vi "Test_WriteValue_InvalidType_Error.vi"(8 "error in (no error)":errorcluster, 11 "TestCase in":refnum<class "TestTerminalVisibilityBinding.lvclass">) -> (0 "error out":errorcluster, 3 "TestCase out":refnum<class "TestTerminalVisibilityBinding.lvclass">)   [LabVIEW 2017, in "TestTerminalVisibilityBinding.lvclass"]
uses:
  TestTerminalVisibilityBinding.lvclass
  Source/Concrete/TerminalVisibilityBinding/TerminalVisibilityBinding.lvclass
  C:/Git/composed-transport/Source/ITransport/ITransport.lvclass
  Source/ITransport/ITransport.lvclass
panel:
  in  "Numeric":dbl
  out "Return Error":errorcluster
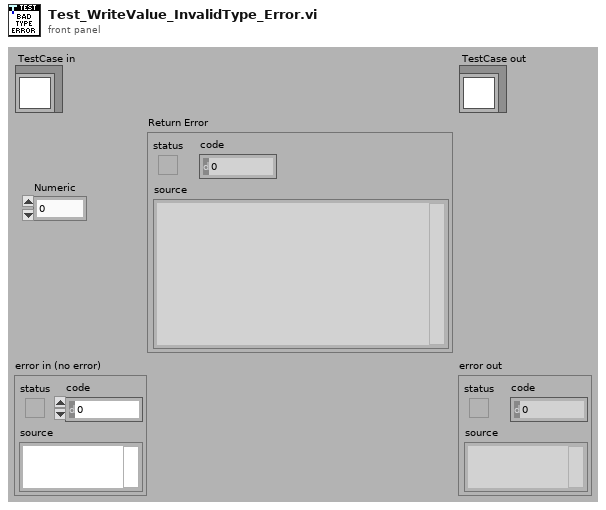
[diagram p1: front panel]
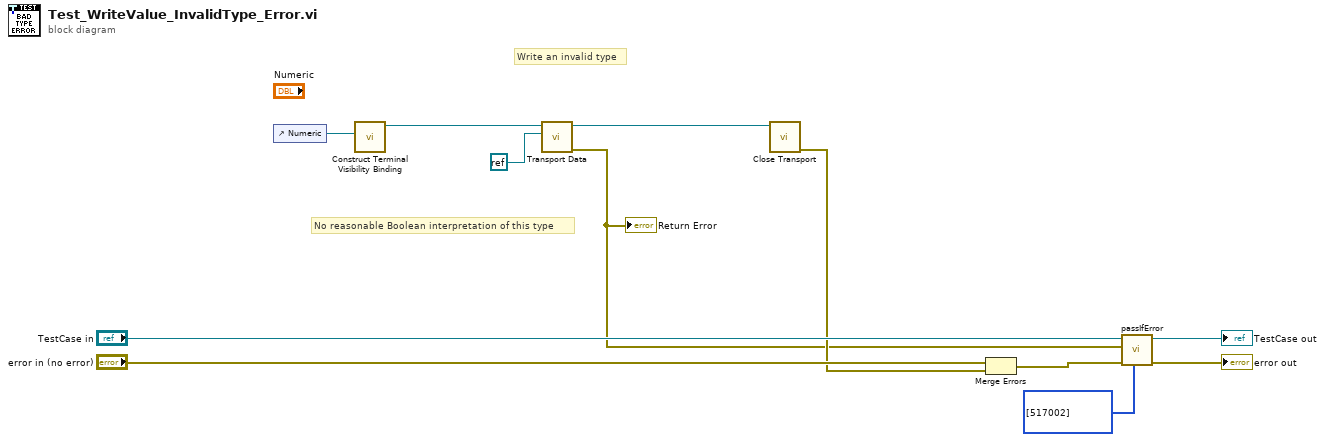
[diagram p0: block diagram]
diagram:
  # "No reasonable Boolean interpretation of this type"
  # "Write an invalid type"
  n1 = control-ref of="Numeric"() -> (w1:refnum<vi>)
  n2 = call "Construct Terminal Visibility Binding.vi"("Ctl Refnum"=w1) -> ("TerminalVisibilityBinding"=w8:refnum<class "TerminalVisibilityBinding.lvclass">)  [unwired: 9 in, 1 out]
  n3 = call "Transport Data.vi"("Value"=refnum<k0> refnum, "ITransport in"=w8) -> ("error out"=w4:errorcluster, "ITransport out"=w6:refnum<class "TerminalVisibilityBinding.lvclass">)  [unwired: 8 in]
  "Return Error" <- w4
  n4 = call-dynamic "Close Transport.vi"("ITransport in"=w6) -> ("error out"=w5:errorcluster)  [unwired: 10 in]
  n5 = Merge Errors("error in (no error)", w5) -> (w7:errorcluster)
  n6 = call-dynamic "passIfError.vi"("passing error codes (default = any error code)"=i32[] [517002], "error in (no error)"=w7, "error"=w4, "TestCase in"="TestCase in") -> ("error out"=→"error out":errorcluster, "TestCase out"=→"TestCase out":refnum<class "TestTerminalVisibilityBinding.lvclass">)  [unwired: 6 in]
